vi "setFPGAReference.vi"(10 "FPGAReference":refnum<k20>, 11 "MyHealthAndStatusReadFIFO in":refnum<class "ModbusPort1ReadFIFO.lvclass">) -> (3 "MyHealthAndStatusReadFIFO out":refnum<class "ModbusPort1ReadFIFO.lvclass">)   [LabVIEW 2015, in "ModbusPort1ReadFIFO.lvclass"]
uses:
  ModbusPort1ReadFIFO.lvclass
  ModbusPort1ReadFIFO.lvclass/ModbusPort1ReadFIFO.ctl
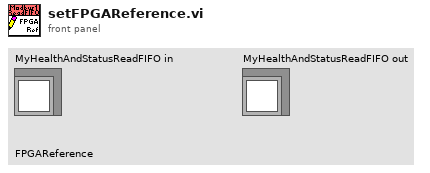
[diagram p1: front panel]
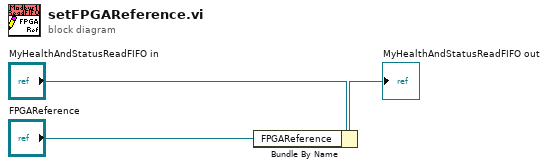
[diagram p0: block diagram]
diagram:
  n1 = Bundle By Name(cluster="MyHealthAndStatusReadFIFO in", "FPGAReference"="FPGAReference") -> (→"MyHealthAndStatusReadFIFO out":refnum<class "ModbusPort1ReadFIFO.lvclass">)
